vi "cblize.vi"   [LabVIEW 2011]
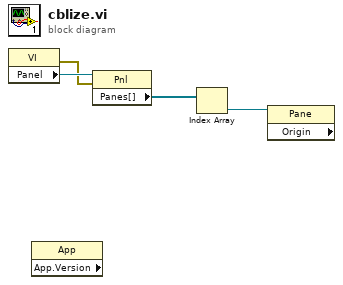
[diagram p0: block diagram]
diagram:
  n1 = property class="VI"() -> (error out=w3:errorcluster, "Panel"=w4:refnum<vi>)  [unwired: 2 in, 1 out]
  n2 = property class="App" props=["App.Version"]() -> ()  [unwired: 2 in, 3 out]
  n3 = property class="Pnl"(reference=w4, error in=w3) -> ("Panes[]"=w2:refnum<vi>[])  [unwired: 2 out]
  n4 = Index Array(array=w2) -> (element=w1:refnum<vi>)  [unwired: 1 in]
  n5 = property class="Pane" props=["Origin"](reference=w1) -> ()  [unwired: 1 in, 3 out]
